vi "Test Write Read.vi"(11 "Test Case In":refnum<class "01_ImageFileIO.lvclass">) -> (0 "error out":errorcluster, 3 "Test Case Out":refnum<class "01_ImageFileIO.lvclass">)   [LabVIEW 2020, in "test.lvlib" / "01_ImageFileIO.lvclass"]
uses:
  01_ImageFileIO.lvclass
  C:/Program Files (x86)/National Instruments/LabVIEW 2026/vi.lib/Astemes/LUnit/Test Case.lvclass
  image/ARGB Colour.ctl
  common/Image Size (Integer).ctl
  01_ImageFileIO.lvclass/01_ImageFileIO.ctl
  <vilib>/Astemes/LUnit/Test Case.lvclass/Test Case.ctl
  image/New Image (ARGB Preallocated).vi/3321fa97-f432-4e1e-8db9-a0df79aed21b.vi
  image/ARGB Colour to U32 Pixel Value.vi
  image/Write Image File (ARGB).vi/9723f547-2605-4a38-b7b5-a8bc0a93fff0.vi
  image/Write PNG File with Alpha.vi/9723f547-2605-4a38-b7b5-a8bc0a93fff0.vi
  image/Read Image File (ARGB).vi/2358f293-6357-4b7a-bec3-c4e4d03be6e5.vi
  <vilib>/Astemes/LUnit/Core/LUnit Test Case/Private/Append Pass Result.vi
  <vilib>/Astemes/LUnit/Core/LUnit Test Case/Private/Append Fail Result.vi
  <vilib>/Astemes/LUnit/Core/LUnit Test Case/Private/Run In UI.vi
  <vilib>/Utility/error.llb/Clear Errors.vi
  <vilib>/Utility/error.llb/Error Cluster From Error Code.vi
  image/image.lvlib
  common/common.lvlib
  <vilib>/Astemes/LUnit/Test Case.lvclass
panel:
  out "Unique Temporary File Path":path
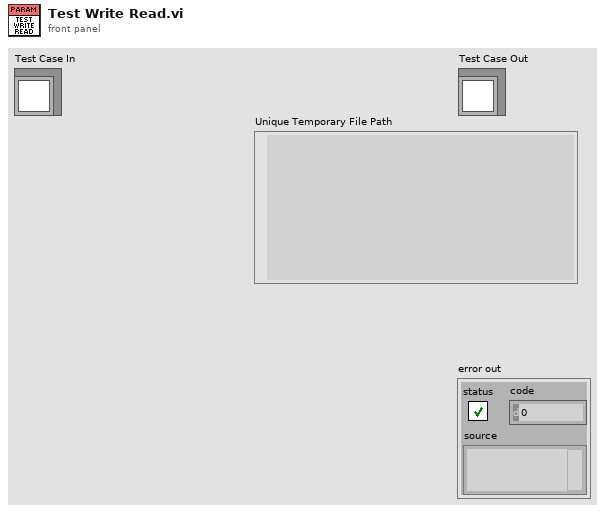
[diagram p1: front panel]
types:
  T1 = typedef "common.lvlib/Image Size (Integer).ctl" = cluster{"Width":u16, "Height":u16}
  T2 = typedef "image.lvlib/ARGB Colour.ctl" = cluster{"Alpha":u8, "RGB":u32}
  T3 = typedef "test.lvlib/01_ImageFileIO.lvclass/Types.ctl" = enum16{"jpeg", "png", "png-alpha", "webp", "tiff"}
  T4 = typedef "image.lvlib/ARGB Image.ctl" = refnum<data-value>
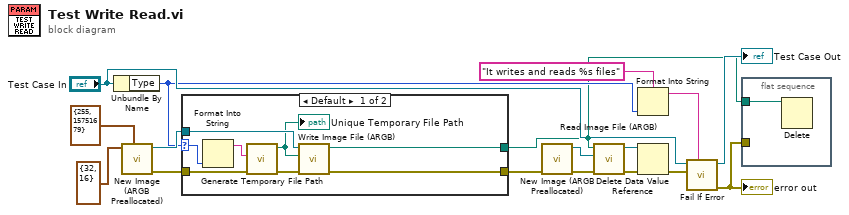
[diagram p0: block diagram]
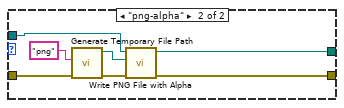
[diagram p2: hidden frame]
diagram:
  n1 = Unbundle By Name("Test Case In") -> ("Type"=w3:T3)
  n2 = call "New Image (ARGB Preallocated).vi"("Colour (Default: Black)"=T2 {"Alpha"=255, "RGB"=15751679}, "Preallocated Image Size (Default: 0,0)"=T1 {"Width"=32, "Height"=16}) -> ("error out"=w12:errorcluster, "ARGB Image"=w13:T4)  [unwired: 8 in]
  n3 = case shown="Default" w3 {
    selector: w3 -> [w18 _]
    tunnel: w13 -> [w25 w32]
    tunnel: w12 -> [w24 w31]
    tunnel: [w21 w28] -> w11
    tunnel: [w20 w27] -> w2
    frame Default {
      n4 = Format Into String(w18) -> (resulting string=w19:string)  [unwired: 3 in, 1 out]
      n5 = call <vilib>:"Generate Temporary File Path.vi"("error in (no error)"=w24, "Temporary File Extension (tmp)"=w19) -> ("error out"=w23:errorcluster, "Unique Temporary File Path"=w22:path)  [unwired: 8 in]
      "Unique Temporary File Path" <- w22
      n6 = call "Write Image File (ARGB).vi"("error in (no error)"=w23, "Filepath in"=w22, "ARGB Image Source in"=w25) -> ("error out"=w21:errorcluster, "Filepath"=w20:path)  [unwired: 7 in]
    }
    frame "png-alpha" {
      n7 = call <vilib>:"Generate Temporary File Path.vi"("error in (no error)"=w31, "Temporary File Extension (tmp)"="png") -> ("error out"=w30:errorcluster, "Unique Temporary File Path"=w29:path)  [unwired: 8 in]
      n8 = call "Write PNG File with Alpha.vi"("error in (no error)"=w30, ".png Filepath in"=w29, "ARGB Image Source in"=w32) -> ("error out"=w28:errorcluster, ".png Filepath"=w27:path)  [unwired: 7 in]
    }
  }
  n9 = call "New Image (ARGB Preallocated).vi"("error in (no error)"=w11) -> ("error out"=w10:errorcluster, "ARGB Image"=w9:T4)  [unwired: 9 in]
  n10 = call "Read Image File (ARGB).vi"("error in (no error)"=w10, "ARGB Image Destination in"=w9, "Filepath"=w2) -> ("error out"=w7:errorcluster, "ARGB Image Destination"=w8:T4)  [unwired: 7 in]
  n11 = Format Into String(format string="It writes and reads %s files", w3) -> (resulting string=w5:string)  [unwired: 2 in, 1 out]
  n12 = Delete Data Value Reference(data value reference=w8, error in=w7) -> (error out=w6:errorcluster)  [unwired: 1 out]
  n13 = call <vilib>:"Fail If Error.vi"("Description"=w5, "Assert error"=w6, "LUnit Test Case In"="Test Case In") -> ("error out"=w1:errorcluster, "LUnit Test Case Out"=→"Test Case Out":refnum<class "01_ImageFileIO.lvclass">)  [unwired: 7 in]
  "error out" <- w1
  n14 = flat-sequence {
    tunnel: w2 -> [w33]
    tunnel: w1 -> [_]
    frame #0 {
      n15 = Delete(path (use dialog)=w33) -> ()  [unwired: 4 in, 3 out]
    }
  }
